vi "make plots.vi"() -> ()   [LabVIEW 2016]
panel:
  in  "Numeric":i32=3
  out "fits 3":cluster{dbl[], dbl[]}[](graph)=[{[-9.0, -8.96, -8.92, -8.88, -8.84, -8.8, -8.76, -8.72, -8.68, -8.64, -8.6, -8.56, -8.52, -8.48, -8.44, -8.4, -8.36, -8.32, -8.28, -8.24, -8.2, -8.16, -8.12, -8.08, -8.04, -8.0, -7.96, -7.92, -7.88, -7.84, -7.8, -7.76, -7.72, -7.68, -7.64, -7.6, -7.5600000000000005, -7.52, -7.48, -7.4399999999999995, -7.4, -7.359999999999999, -7.32, -7.28, -7.24, -7.2, -7.16, -7.12, -7.08, -7.04, -7.0, -6.96, -6.92, -6.88, -6.84, -6.8, -6.76, -6.72, -6.68, -6.640000000000001, -6.6, -6.5600000000000005, -6.52, -6.48, -6.4399999999999995, -6.4, -6.359999999999999, -6.32, -6.279999999999999, -6.24, -6.199999999999999, -6.16, -6.12, -6.08, -6.04, -6.0, -5.96, -5.92, -5.88, -5.84, -5.8, -5.76, -5.72, -5.68, -5.640000000000001, -5.6, -5.5600000000000005, -5.52, -5.48, -5.4399999999999995, -5.4, -5.359999999999999, -5.32, -5.279999999999999, -5.24, -5.199999999999999, -5.16, -5.12, -5.08, -5.04, -5.0, -4.96, -4.92, -4.88, -4.84, -4.8, -4.76, -4.72, -4.68, -4.64, -4.6, -4.56, -4.52, -4.4799999999999995, -4.4399999999999995, -4.3999999999999995, -4.36, -4.32, -4.28, -4.24, -4.2, -4.16, -4.12, -4.08, -4.04, -4.0, -3.96, -3.92, -3.88, -3.84, -3.8, -3.76, -3.7199999999999998, -3.6799999999999997, -3.6399999999999997, -3.5999999999999996, -3.5599999999999996, -3.5199999999999996, -3.4799999999999995, -3.4399999999999995, -3.3999999999999995, -3.3600000000000003, -3.3200000000000003, -3.2800000000000002, -3.24, -3.2, -3.16, -3.12, -3.08, -3.04], [0.0, 0.5298858238579937, 0.5291899826987614, 0.5287099077407282, 0.5286651463233265, 0.5279979941515467, 0.527816733946416, 0.5270333124515219, 0.5271761948115984, 0.5266780264585993, 0.5262085664235602, 0.5256436334900743, 0.5248320207172359, 0.5243795083942617, 0.5240650115761005, 0.5232398840351181, 0.5304366203739485, 0.522161059460385, 0.5218481873140289, 0.5209133415901583, 0.5206236932263532, 0.520104035495158, 0.5191505915843438, 0.5186928417610543, 0.517960081588197, 0.5200948863263483, 0.5182633246145715, 0.5174906303778686, 0.5165277359827113, 0.5152937136447644, 0.5140946565141463, 0.5126408752904663, 0.5115306669025806, 0.5103482627248314, 0.5094466289571671, 0.5081094392666907, 0.5066931811698935, 0.5054908922866449, 0.5047226581118076, 0.5016953936282248, 0.49843458738733754, 0.49663027130158727, 0.4946057293670207, 0.4985945435419704, 0.49746003738898786, 0.4891753852627261, 0.48690406700305205, 0.48529177332965273, 0.48308323706174605, 0.48115808497444, 0.4799642589002078, 0.4780290185603138, 0.47588905272811666, 0.47431398370926936, 0.4728943305948261, 0.47075772072806316, 0.46916334917270475, 0.4822810112630788, 0.4654000236510049, 0.4641607539446438, 0.46248086472826755, 0.46054805804273774, 0.45897428953992314, 0.4574671594283139, 0.45564135368614733, 0.4539473656167584, 0.45239624515756577, 0.4508163573779298, 0.44921094843567183, 0.4478707099152407, 0.4459923788867531, 0.4445385566875663, 0.44300169432075537, 0.441508137100753, 0.44005791884245965, 0.4387905856198324, 0.4372202186619696, 0.43574250042173523, 0.43441586934356674, 0.43241506901963306, 0.4310831198697872, 0.42999312229282816, 0.42875526714172313, 0.42717783268743564, 0.42605246735742613, 0.4247507737494975, 0.42343391087618804, 0.42235167459147543, 0.4206700914991393, 0.4193026904238367, 0.4180852226827774, 0.4163945769922073, 0.41490706113338754, 0.41331561343133466, 0.4117539982838646, 0.4103247286249982, 0.40873696369120605, 0.40704040345483994, 0.40541788189249234, 0.40385930727039454, 0.402187517297513, 0.4004362177171245, 0.3987255497740591, 0.39708616055882323, 0.3953736068707004, 0.39349641572273475, 0.3919015869096145, 0.390438742318364, 0.3885881132973352, 0.3868683346494929, 0.38547598648350445, 0.3834413713112424, 0.38214365998473726, 0.3805632151703166, 0.3788854018278639, 0.3774107112339481, 0.3756002968146913, 0.37388690943925335, 0.3723744077607701, 0.37113329480803064, 0.36956468793175234, 0.3680162212839035, 0.36636592786395644, 0.3648356074221625, 0.36341479480339794, 0.3619428520810152, 0.36026082646776764, 0.35875669731819526, 0.3575269519142971, 0.3560382047266694, 0.35456612001527854, 0.3531009626285239, 0.35178662821112916, 0.3503833129067078, 0.3491835998154125, 0.347748266235487, 0.34643158821457526, 0.34471954346037154, 0.3433882218639101, 0.3420730817916927, 0.34040628244761456, 0.3393146838556441, 0.3377886197110437, 0.3365900730641488, 0.3354669600271455, 0.3342671382363059, 0.3330043571764805, 0.3313439990334121, 0.3303696704380371, 0.3292207819288466]}, ...(150 in all)]
  in  "fits 2":cluster{dbl[], dbl[]}[](graph)=[{[-9.0, -8.96, -8.92, -8.88, -8.84, -8.8, -8.76, -8.72, -8.68, -8.64, -8.6, -8.56, -8.52, -8.48, -8.44, -8.4, -8.36, -8.32, -8.28, -8.24, -8.2, -8.16, -8.12, -8.08, -8.04, -8.0, -7.96, -7.92, -7.88, -7.84, -7.8, -7.76, -7.72, -7.68, -7.64, -7.6, -7.5600000000000005, -7.52, -7.48, -7.4399999999999995, -7.4, -7.359999999999999, -7.32, -7.28, -7.24, -7.2, -7.16, -7.12, -7.08, -7.04, -7.0, -6.96, -6.92, -6.88, -6.84, -6.8, -6.76, -6.72, -6.68, -6.640000000000001, -6.6, -6.5600000000000005, -6.52, -6.48, -6.4399999999999995, -6.4, -6.359999999999999, -6.32, -6.279999999999999, -6.24, -6.199999999999999, -6.16, -6.12, -6.08, -6.04, -6.0, -5.96, -5.92, -5.88, -5.84, -5.8, -5.76, -5.72, -5.68, -5.640000000000001, -5.6, -5.5600000000000005, -5.52, -5.48, -5.4399999999999995, -5.4, -5.359999999999999, -5.32, -5.279999999999999, -5.24, -5.199999999999999, -5.16, -5.12, -5.08, -5.04, -5.0, -4.96, -4.92, -4.88, -4.84, -4.8, -4.76, -4.72, -4.68, -4.64, -4.6, -4.56, -4.52, -4.4799999999999995, -4.4399999999999995, -4.3999999999999995, -4.36, -4.32, -4.28, -4.24, -4.2, -4.16, -4.12, -4.08, -4.04, -4.0, -3.96, -3.92, -3.88, -3.84, -3.8, -3.76, -3.7199999999999998, -3.6799999999999997, -3.6399999999999997, -3.5999999999999996, -3.5599999999999996, -3.5199999999999996, -3.4799999999999995, -3.4399999999999995, -3.3999999999999995, -3.3600000000000003, -3.3200000000000003, -3.2800000000000002, -3.24, -3.2, -3.16, -3.12, -3.08, -3.04], [0.0, 0.5298858238579937, 0.5291899826987614, 0.5287099077407282, 0.5286651463233265, 0.5279979941515467, 0.527816733946416, 0.5270333124515219, 0.5271761948115984, 0.5266780264585993, 0.5262085664235602, 0.5256436334900743, 0.5248320207172359, 0.5243795083942617, 0.5240650115761005, 0.5232398840351181, 0.5304366203739485, 0.522161059460385, 0.5218481873140289, 0.5209133415901583, 0.5206236932263532, 0.520104035495158, 0.5191505915843438, 0.5186928417610543, 0.517960081588197, 0.5200948863263483, 0.5182633246145715, 0.5174906303778686, 0.5165277359827113, 0.5152937136447644, 0.5140946565141463, 0.5126408752904663, 0.5115306669025806, 0.5103482627248314, 0.5094466289571671, 0.5081094392666907, 0.5066931811698935, 0.5054908922866449, 0.5047226581118076, 0.5016953936282248, 0.49843458738733754, 0.49663027130158727, 0.4946057293670207, 0.4985945435419704, 0.49746003738898786, 0.4891753852627261, 0.48690406700305205, 0.48529177332965273, 0.48308323706174605, 0.48115808497444, 0.4799642589002078, 0.4780290185603138, 0.47588905272811666, 0.47431398370926936, 0.4728943305948261, 0.47075772072806316, 0.46916334917270475, 0.4822810112630788, 0.4654000236510049, 0.4641607539446438, 0.46248086472826755, 0.46054805804273774, 0.45897428953992314, 0.4574671594283139, 0.45564135368614733, 0.4539473656167584, 0.45239624515756577, 0.4508163573779298, 0.44921094843567183, 0.4478707099152407, 0.4459923788867531, 0.4445385566875663, 0.44300169432075537, 0.441508137100753, 0.44005791884245965, 0.4387905856198324, 0.4372202186619696, 0.43574250042173523, 0.43441586934356674, 0.43241506901963306, 0.4310831198697872, 0.42999312229282816, 0.42875526714172313, 0.42717783268743564, 0.42605246735742613, 0.4247507737494975, 0.42343391087618804, 0.42235167459147543, 0.4206700914991393, 0.4193026904238367, 0.4180852226827774, 0.4163945769922073, 0.41490706113338754, 0.41331561343133466, 0.4117539982838646, 0.4103247286249982, 0.40873696369120605, 0.40704040345483994, 0.40541788189249234, 0.40385930727039454, 0.402187517297513, 0.4004362177171245, 0.3987255497740591, 0.39708616055882323, 0.3953736068707004, 0.39349641572273475, 0.3919015869096145, 0.390438742318364, 0.3885881132973352, 0.3868683346494929, 0.38547598648350445, 0.3834413713112424, 0.38214365998473726, 0.3805632151703166, 0.3788854018278639, 0.3774107112339481, 0.3756002968146913, 0.37388690943925335, 0.3723744077607701, 0.37113329480803064, 0.36956468793175234, 0.3680162212839035, 0.36636592786395644, 0.3648356074221625, 0.36341479480339794, 0.3619428520810152, 0.36026082646776764, 0.35875669731819526, 0.3575269519142971, 0.3560382047266694, 0.35456612001527854, 0.3531009626285239, 0.35178662821112916, 0.3503833129067078, 0.3491835998154125, 0.347748266235487, 0.34643158821457526, 0.34471954346037154, 0.3433882218639101, 0.3420730817916927, 0.34040628244761456, 0.3393146838556441, 0.3377886197110437, 0.3365900730641488, 0.3354669600271455, 0.3342671382363059, 0.3330043571764805, 0.3313439990334121, 0.3303696704380371, 0.3292207819288466]}, ...(150 in all)]
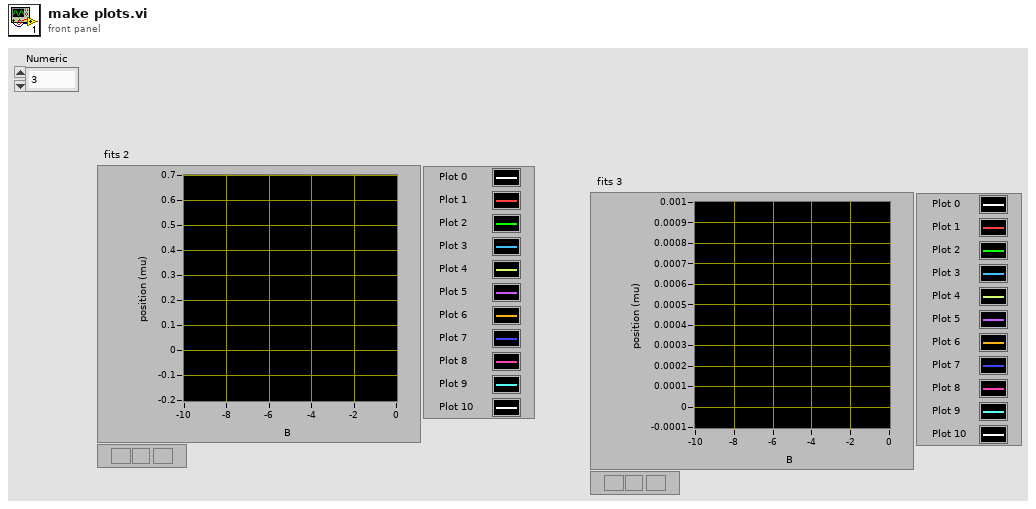
[diagram p1: front panel]
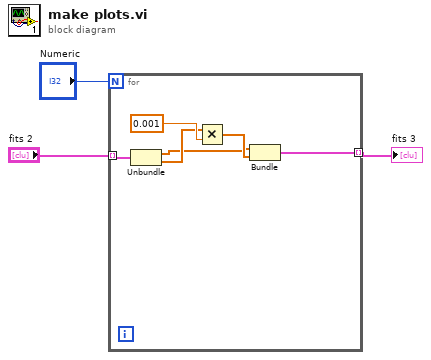
[diagram p0: block diagram]
diagram:
  n1 = for {
    N: "Numeric" -> [_]
    tunnel: "fits 2" -> [w9] mode=indexing
    tunnel: [w7] -> w2 mode=indexing
    n2 = Unbundle(w9) -> (w4:dbl[], w6:dbl[])
    n3 = Multiply(x=w6, y=0.001) -> (x*y=w5:dbl[])
    n4 = Bundle(w4, w5) -> (w7:cluster{dbl[], dbl[]})  [unwired: 1 in]
  }
  "fits 3" <- w2
